vi "ReadCapacitanceBuffers.vi"(8 "error in (no error)":errorcluster, 10 "Status":refnum<vi>, 11 "VISA Refnum in":refnum<visa-resource-name>) -> (0 "error out":errorcluster, 1 "status":bool, 3 "CapacitanceInfos":T1[](array[typedef]))   [LabVIEW 2020]
uses:
  CapacitanceRecord.ctl
  Keithley 2600 Series/Keithley 2600 Series.lvlib
panel:
  out "error out 3":errorcluster
  in  "VISA resource name":refnum<visa-resource-name>="Keithley_2636A"
  out "Array":string[](array[string])
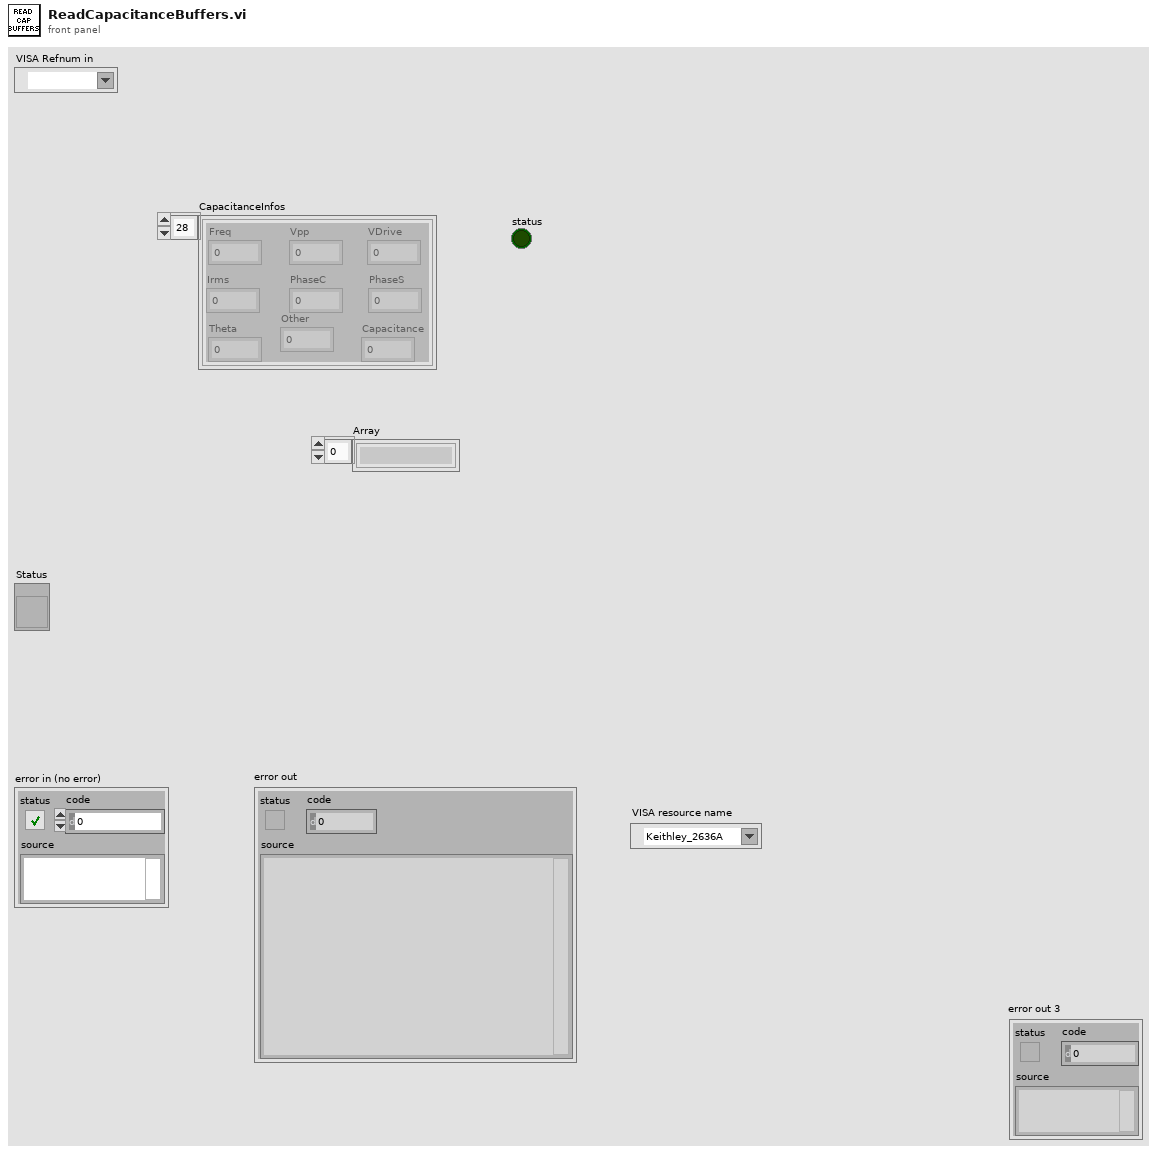
[diagram p1: front panel]
types:
  T1 = typedef "CapacitanceRecord.ctl" = cluster{"Freq":dbl, "Vpp":dbl, "PhaseS":dbl, "Irms":dbl, "PhaseC":dbl, "Theta":dbl, "VDrive":dbl, "Capacitance":dbl, "Other":dbl}
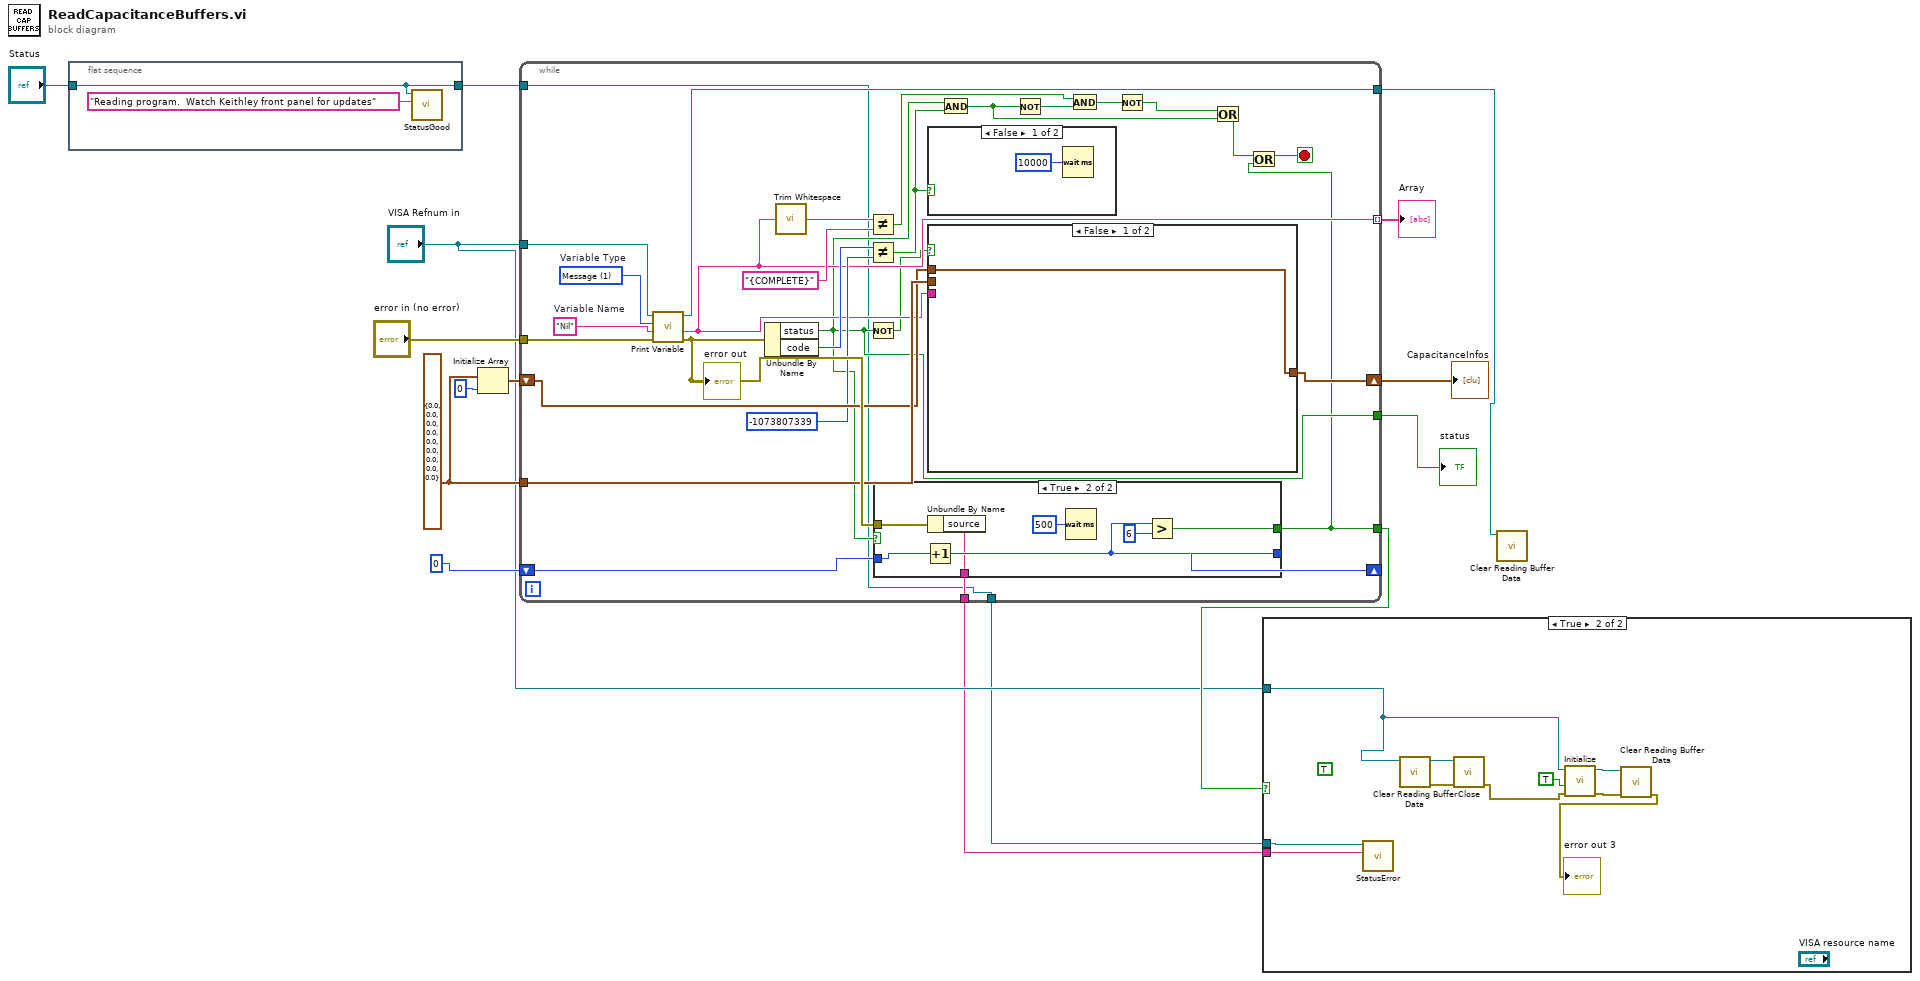
[diagram p0: block diagram]
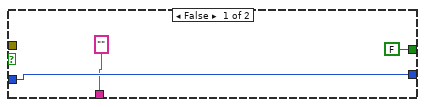
[diagram p4: hidden frame]
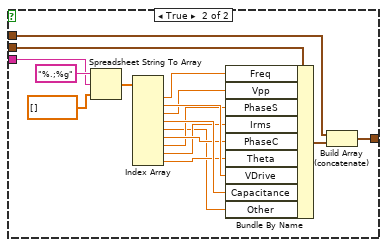
[diagram p5: hidden frame]
diagram:
  w12 = T1 {"Freq"=0.0, "Vpp"=0.0, "PhaseS"=0.0, "Irms"=0.0, "PhaseC"=0.0, "Theta"=0.0, "VDrive"=0.0, "Capacitance"=0.0, "Other"=0.0} ("cluster")
  n1 = flat-sequence {
    tunnel: "Status" -> [w16]
    tunnel: [w16] -> w8
    frame #0 {
      n2 = call "StatusGood.vi"("Text.Text"="Reading program.  Watch Keithley front panel for updates", "String in"=w16) -> ()  [unwired: 10 in]
    }
  }
  n3 = Initialize Array(w12, 0 ("dimension size")) -> (w11:T1[])
  n4 = while {
    tunnel: "VISA Refnum in" -> [w20]
    tunnel: "error in (no error)" -> [w27]
    tunnel: [w44] -> w3
    shift-right: [w37] -> w13
    shift-left: w11 -> [w35]
    tunnel: w8 -> [w18]
    tunnel: w12 -> [w36]
    tunnel: [w29] -> w10 mode=indexing
    tunnel: [w25] -> w7
    shift-right: [w23] -> _
    shift-left: 0 -> [w24]
    tunnel: [w21] -> w5
    tunnel: [w19] -> w2
    tunnel: [w18] -> w1
    stop <- w22 stop-if-true
    w46 = 1 items=["Number", "Message"]  # Variable Type
    w45 = "Nil"  # Variable Name
    n5 = call "Print Variable.vi"("error in (no error)"=w27, "Variable Name"=w45, "Variable Type (0: Number)"=w46, "VISA resource name"=w20) -> ("error out"=w38:errorcluster, "Message"=w29:string, "VISA resource name out"=w44:refnum<visa-resource-name>)  [unwired: 4 in, 1 out]
    "error out" <- w38
    n6 = Unbundle By Name(w38) -> ("status"=w25:bool, "code"=w34:i32)
    n7 = call <vilib>:"Trim Whitespace.vi"("string"=w29) -> ("trimmed string"=w43:string)  [unwired: 1 in]
    n8 = Not Equal?(x=w43, y="{COMPLETE}") -> (x != y?=w41:bool)
    n9 = Not Equal?(x=w34, y=-1073807339) -> (x != y?=w26:bool)
    n10 = Not(x=w25) -> (.not. x?=w28:bool)
    n11 = case shown="True" w25 {
      tunnel: w38 -> [_ w57]
      tunnel: w24 -> [w50 w56]
      tunnel: [w50 w54] -> w23
      tunnel: [FALSE w52] -> w21
      tunnel: ["" ("source") w51] -> w19
      frame False {
      }
      frame True {
        n12 = Increment(x=w56) -> (x+1=w54:i32)
        n13 = Unbundle By Name(w57) -> ("source"=w51:string)
        n14 = Wait (ms)(milliseconds to wait=u32 500) -> ()  [unwired: 1 out]
        n15 = Greater?(x=w54, y=6) -> (0:w52:bool)
      }
    }
    n16 = case shown="False" w26 {
      frame False {
        n17 = Wait (ms)(milliseconds to wait=u32 10000) -> ()  [unwired: 1 out]
      }
      frame True {
      }
    }
    n18 = case shown="False" w28 {
      tunnel: w29 -> [_ w73]
      tunnel: w35 -> [w58 w72]
      tunnel: [w58 w71] -> w37
      tunnel: w36 -> [_ w70]
      frame False {
      }
      frame True {
        n19 = Spreadsheet String To Array(format string="%.;%g", spreadsheet string=w73, array type (2D Dbl)=dbl[] []) -> (array=w68:dbl[])  [unwired: 1 in]
        n20 = Index Array(array=w68) -> (element #1=w67:dbl, element #2=w66:dbl, element #3=w65:dbl, element #4=w64:dbl, element #5=w59:dbl, element #6=w63:dbl, element #7=w62:dbl, element #8=w61:dbl, element #9=w60:dbl)  [unwired: 9 in]
        n21 = Bundle By Name(cluster=w70, "Freq"=w67, "Vpp"=w65, "PhaseS"=w62, "Irms"=w61, "PhaseC"=w63, "Theta"=w60, "VDrive"=w66, "Capacitance"=w64, "Other"=w59) -> (w69:T1)
        n22 = Build Array (concatenate)(w72, w69) -> (w71:T1[])
      }
    }
    n23 = And(x=w25, y=w26) -> (x .and. y?=w31:bool)
    n24 = Not(x=w31) -> (.not. x?=w30:bool)
    n25 = And(x=w41, y=w30) -> (x .and. y?=w32:bool)
    n26 = Not(x=w32) -> (.not. x?=w40:bool)
    n27 = Or(x=w40, y=w31) -> (x .or. y?=w39:bool)
    n28 = Or(x=w39, y=w21) -> (x .or. y?=w22:bool)
  }
  "CapacitanceInfos" <- w13
  "Array" <- w10
  "status" <- w7
  n29 = case shown="True" w5 {
    tunnel: "VISA Refnum in" -> [_ w78]
    tunnel: w2 -> [_ w77]
    tunnel: w1 -> [_ w76]
    frame False {
    }
    frame True {
      (unwired) TRUE ("Reset (True)")
      n30 = call "StatusError.vi"("Text.Text"=w77, "String in"=w76) -> ()  [unwired: 10 in]
      n31 = call "Clear Reading Buffer Data.vi"("VISA resource name"=w78) -> ("error out"=w85:errorcluster, "VISA resource name out"=w84:refnum<visa-resource-name>)  [unwired: 9 in]
      n32 = call "Close.vi"("error in (no error)"=w85, "VISA resource name"=w84) -> ("error out"=w80:errorcluster)  [unwired: 9 in]
      n33 = call "Initialize.vi"("error in (no error)"=w80, "Reset (True)"=TRUE, "VISA resource name"=w78) -> ("error out"=w81:errorcluster, "VISA resource name out"=w82:refnum<visa-resource-name>)  [unwired: 7 in]
      n34 = call "Clear Reading Buffer Data.vi"("error in (no error)"=w81, "VISA resource name"=w82) -> ("error out"=→"error out 3":errorcluster)  [unwired: 8 in, 1 out]
    }
  }
  n35 = call "Clear Reading Buffer Data.vi"("VISA resource name"=w3) -> ()  [unwired: 9 in, 2 out]
